vi "Example 05b - Large Arrays.vi"() -> ()   [LabVIEW 2020]
uses:
  Lua for LabVIEW/Lua/Lua.lvclass
panel:
  out "» Mem Bytes (after gc)":i64 format="%.1p"
  out "» Mem Bytes (after release my_array)":i64 format="%.1p"
  out "» Mem Bytes (after array initialization)":i64 format="%.1p"
  out "» Mem Bytes (before array initialization)":i64 format="%.1p"
  in  "length":i64=5
  in  "offset":i64=30000
  out "#my_array":i64
  out "subset":i64[](array[numeric])
  out "error out":errorcluster
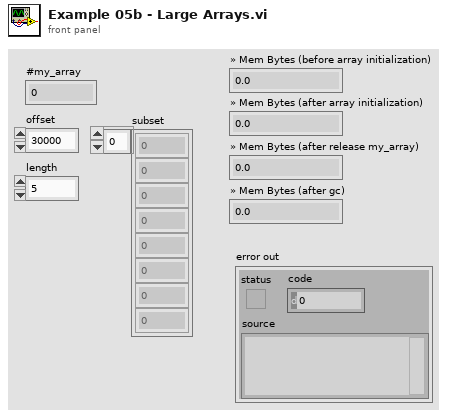
[diagram p1: front panel]
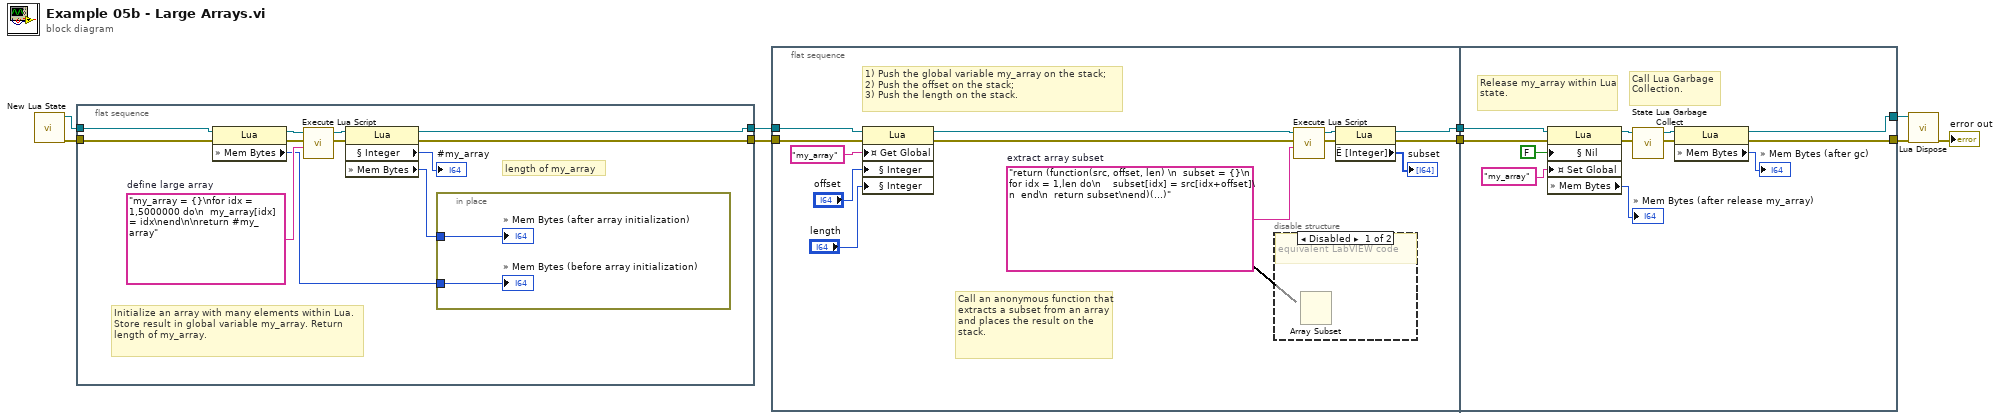
[diagram p0: block diagram]
diagram:
  n1 = call "New Lua State.vi"() -> ("error out"=w9:errorcluster, "Lua out"=w5:refnum<class "Lua.lvclass">)  [unwired: 10 in]
  n2 = flat-sequence {
    tunnel: w9 -> [w13]
    tunnel: w5 -> [w21]
    tunnel: [w18] -> w4
    tunnel: [w17] -> w3
    frame #0 {
      w16 = "my_array = {}\nfor idx = 1,5000000 do\n  my_array[idx] = idx\nend\n\nreturn #my_array"  # define large array
      # "length of my_array"
      # "Initialize an array with many elements within Lua. Store result in global variable my_array. Return length of my_array."
      n3 = property class="Lua"(reference=w21, error in=w13) -> (reference out=w14:refnum<class "Lua.lvclass">, error out=w12:errorcluster, "» Mem Bytes"=w11:i64)
      n4 = call-dynamic "Execute Lua Script.vi"("lua script"=w16, "error in (no error)"=w12, "Lua in"=w14) -> ("error out"=w15:errorcluster, "Lua out"=w20:refnum<class "Lua.lvclass">)  [unwired: 7 in]
      n5 = property class="Lua"(reference=w20, error in=w15) -> (reference out=w18:refnum<class "Lua.lvclass">, error out=w17:errorcluster, "§ Integer"=→"#my_array":i64, "» Mem Bytes"=w10:i64)
      n6 = in-place {
        in-place-border: w11 -> [w23]
        in-place-border: w10 -> [w22]
        "» Mem Bytes (before array initialization)" <- w23
        "» Mem Bytes (after array initialization)" <- w22
      }
    }
  }
  n7 = flat-sequence {
    tunnel: w4 -> [w32]
    tunnel: w3 -> [w30]
    tunnel: [w36] -> w2
    tunnel: [w35] -> w1
    tunnel: [w39] -> w7
    tunnel: [w40] -> w8
    tunnel: w2 -> [w48]
    tunnel: w1 -> [w46]
    frame #0 {
      w26 = "return (function(src, offset, len) \n  subset = {}\n  for idx = 1,len do\n    subset[idx] = src[idx+offset]\n  end\n  return subset\nend)(...)"  # extract array subset
      # "Call an anonymous function that extracts a subset from an array and places the result on the stack."
      # "1) Push the global variable my_array on the stack;\n2) Push the offset on the stack;\n3) Push the length on the stack."
      n8 = property class="Lua"(reference=w32, error in=w30, "¤ Get Global"="my_array" ("§ String"), "§ Integer"="offset", "§ Integer"="length") -> (reference out=w31:refnum<class "Lua.lvclass">, error out=w25:errorcluster)
      n9 = disable-structure shown="Disabled" {
        frame Disabled {
          # "equivalent LabVIEW code"
          n10 = Array Subset "Array Subset"() -> ()  [unwired: 3 in, 1 out]
        }
        frame Enabled {
        }
      }
      n11 = call-dynamic "Execute Lua Script.vi"("lua script"=w26, "error in (no error)"=w25, "Lua in"=w31) -> ("error out"=w24:errorcluster, "Lua out"=w33:refnum<class "Lua.lvclass">)  [unwired: 7 in]
      n12 = property class="Lua"(reference=w33, error in=w24) -> (reference out=w36:refnum<class "Lua.lvclass">, error out=w35:errorcluster, "Ё [Integer]"=→"subset":i64[])
    }
    frame #1 {
      # "Call Lua Garbage Collection."
      # "Release my_array within Lua state."
      n13 = property class="Lua"(reference=w48, error in=w46, "§ Nil"=FALSE, "¤ Set Global"="my_array") -> (reference out=w47:refnum<class "Lua.lvclass">, error out=w42:errorcluster, "» Mem Bytes"=→"» Mem Bytes (after release my_array)":i64)
      n14 = call-dynamic "State Lua Garbage Collect.vi"("error in (no error)"=w42, "Lua in"=w47) -> ("error out"=w38:errorcluster, "Lua out"=w41:refnum<class "Lua.lvclass">)  [unwired: 7 in, 1 out]
      n15 = property class="Lua"(reference=w41, error in=w38) -> (reference out=w40:refnum<class "Lua.lvclass">, error out=w39:errorcluster, "» Mem Bytes"=→"» Mem Bytes (after gc)":i64)
    }
  }
  n16 = call-dynamic "Lua Dispose.vi"("error in (no error)"=w7, "Lua in"=w8) -> ("error out"=→"error out":errorcluster)  [unwired: 9 in]
